vi "spustanje na 2MHz.vi"(10 "Filtered Signal 2":dynamicdata(waveform), 11 "Filtered Signal":dynamicdata(waveform)) -> (1 "IQ 2MHz  spektar":dynamicdata(graph), 2 "IQ 2MHz":dynamicdata(graph), 3 "I grana 2MHz":dynamicdata(graph), 4 "Q grana 2MHz":dynamicdata(graph))   [LabVIEW 2018]
uses:
  <vilib>/express/express analysis/Spectral/Block/exnSpectralBlock spectral measurements RMS poly.vi
  <vilib>/express/express analysis/Spectral/XNode/ExpressSpectralMeasurementsBlockNode.xnode
  <vilib>/express/express analysis/Spectral/Block/exnSpectralBlock spectral measurements RMS DDT.vi
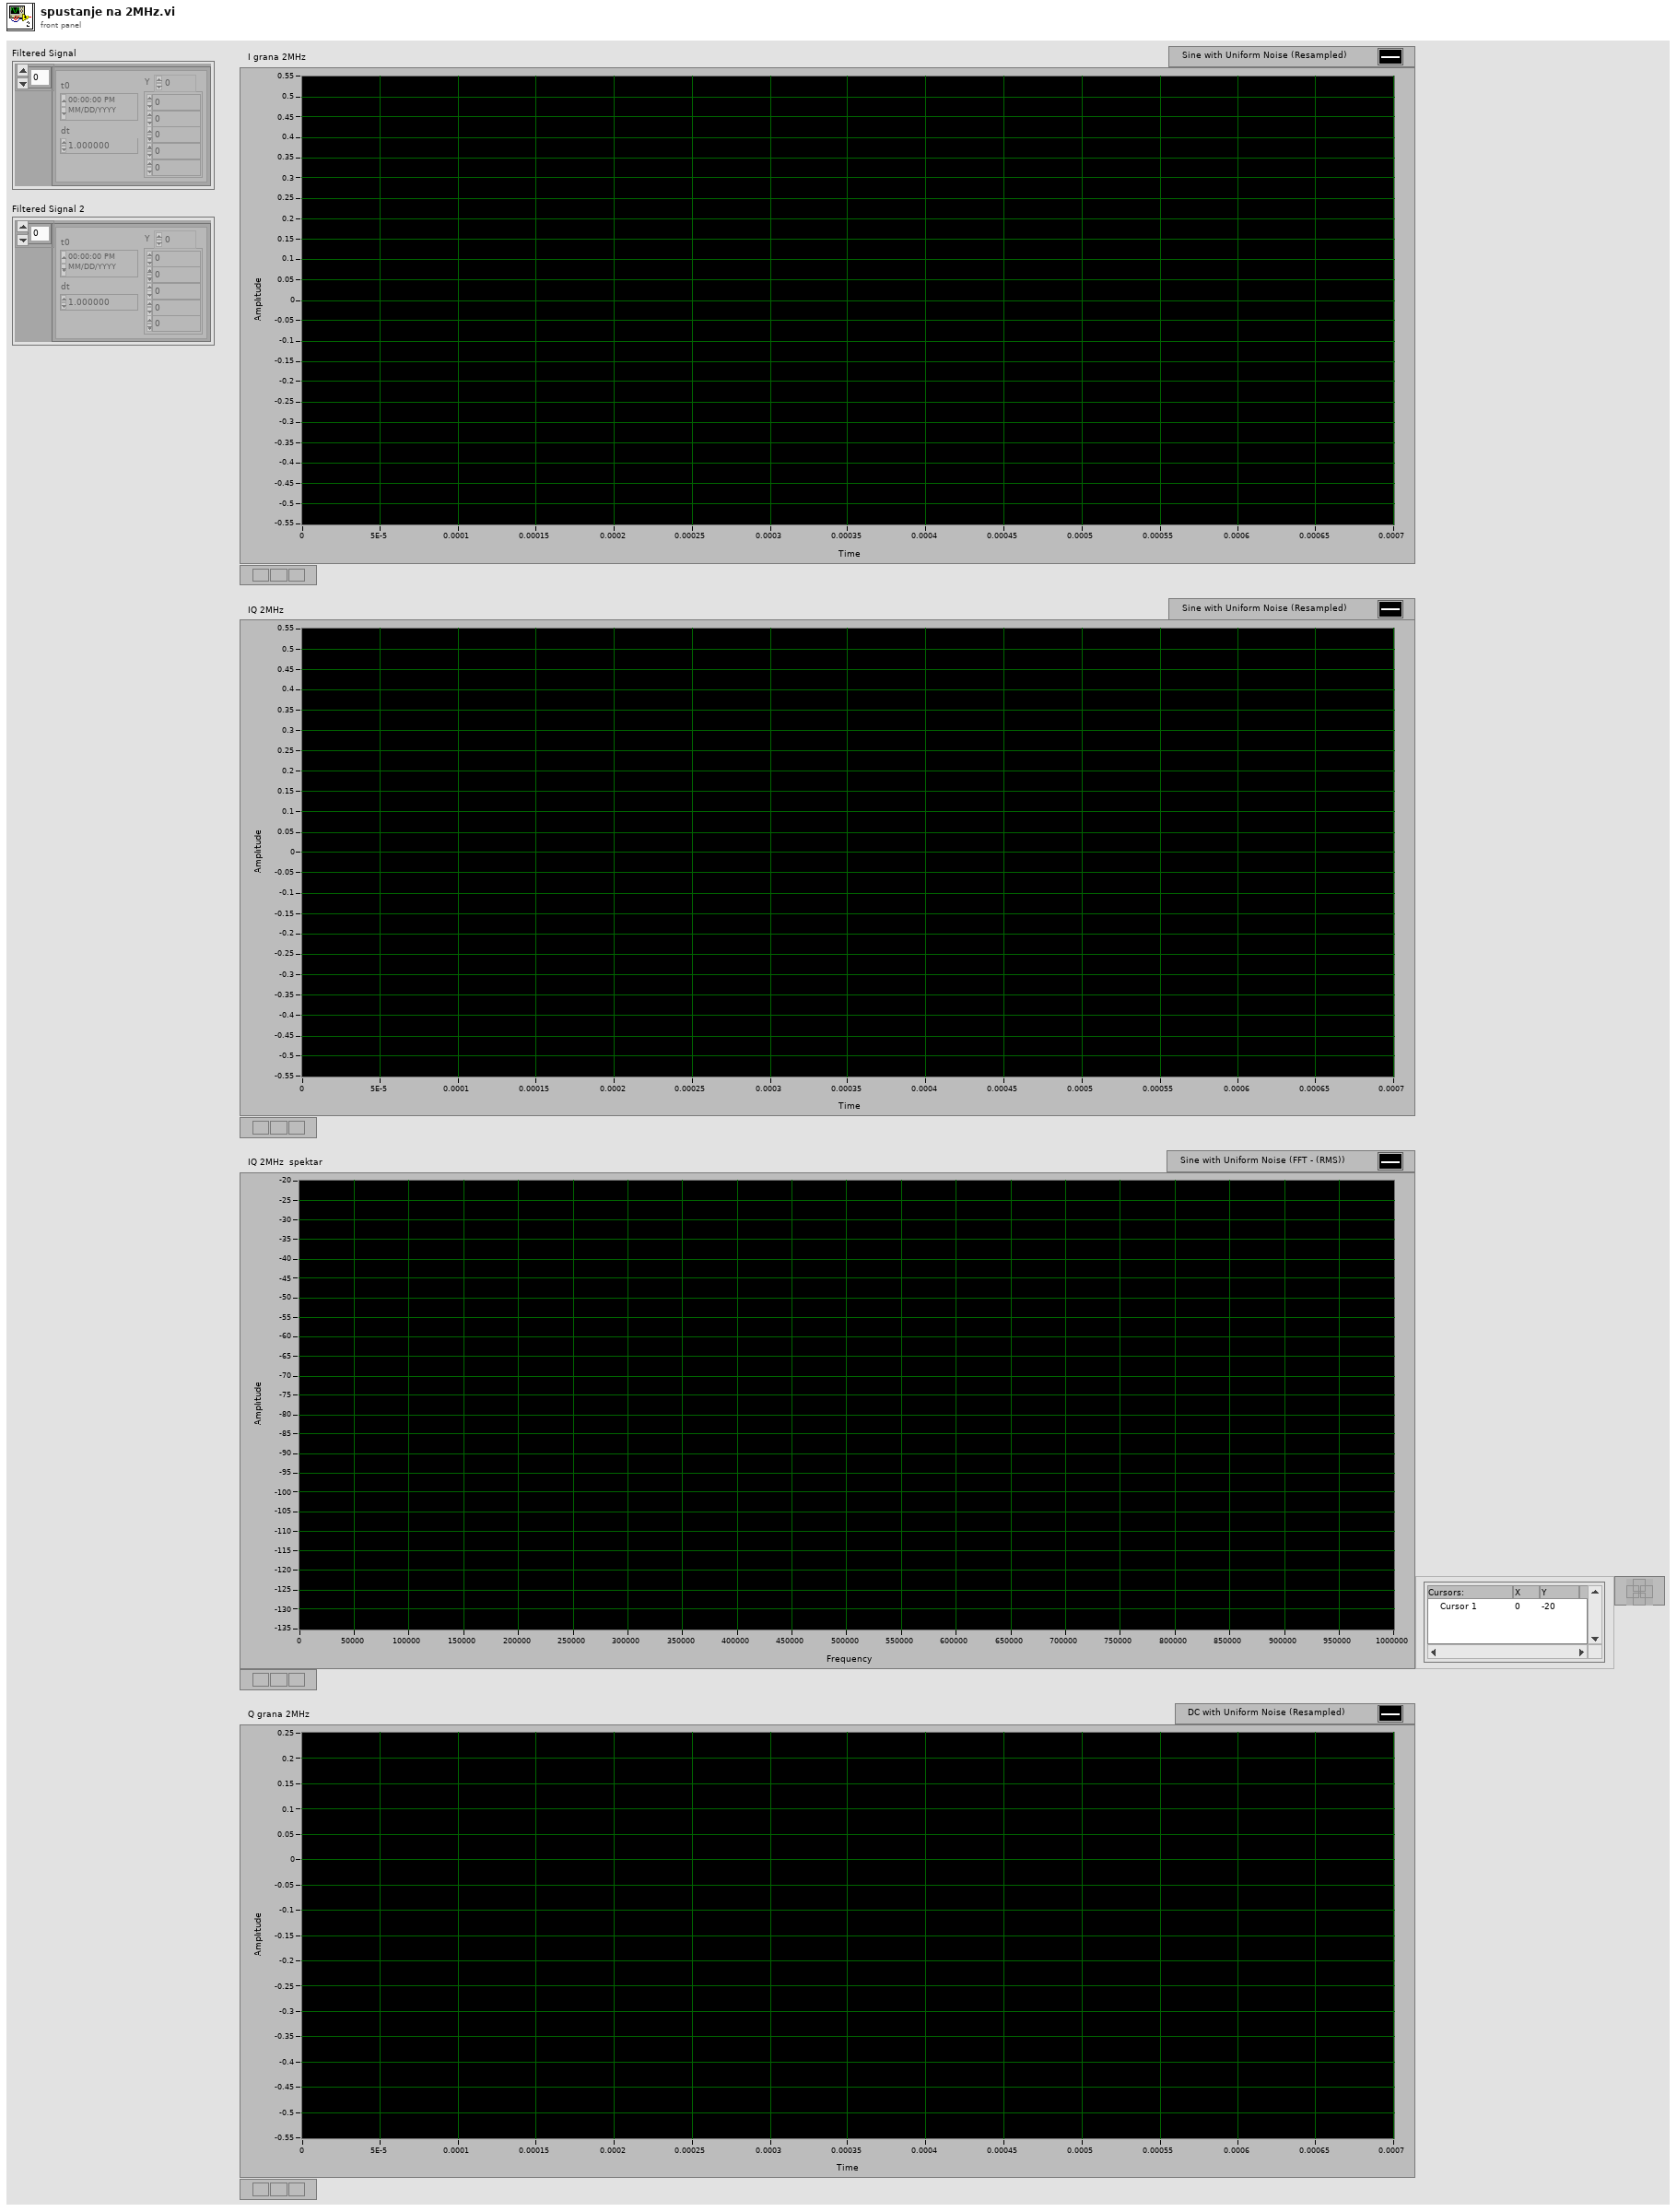
[diagram p1: front panel]
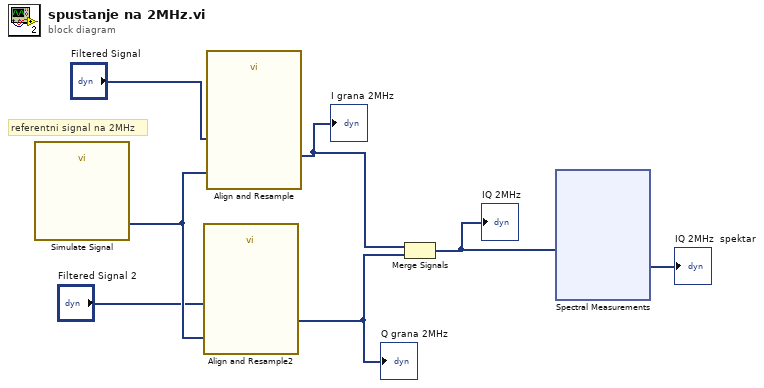
[diagram p0: block diagram]
diagram:
  # "referentni signal na 2MHz"
  n1 = call "Simulate Signal"() -> ("Sine"=w2:dynamicdata)  [unwired: 14 in, 1 out]
  n2 = call "Align and Resample2"("Reference Signal"=w2, "Signals"="Filtered Signal 2") -> ("Resampled Signals"=w4:dynamicdata)  [unwired: 7 in, 2 out]
  "Q grana 2MHz" <- w4
  n3 = call "Align and Resample"("Reference Signal"=w2, "Signals"="Filtered Signal") -> ("Resampled Signals"=w3:dynamicdata)  [unwired: 7 in, 2 out]
  "I grana 2MHz" <- w3
  n4 = Merge Signals(w3, w4) -> (w5:dynamicdata)
  "IQ 2MHz" <- w5
  n5 = xnode "Spectral Measurements"("Signals"=w5) -> ("FFT - (RMS)"=→"IQ 2MHz  spektar":dynamicdata)  [unwired: 1 in, 2 out]
